vi "TwoCameraDisplayPanel.vi"() -> ()   [LabVIEW 2011]
uses:
  MvLVLib/MvCameraControl.lvlib
  MvLVLib/VIs/CreateGigEHandle.vi
  MvLVLib/VIs/CreateU3VHandle.vi
  <vilib>/picture/picture.llb/imagedata.ctl
panel:
  in  "image data 2":T1 caption="图像数据"
  in  "Rectangle 2":T2
  out "pFrameInfoEx out 2":T3
  in  "pConvertInfo In 2":T4
  out "nWidth 2":u32
  out "nHeight 2":u32
  out "PayloadSize 2":u32
  out "PixelFormat 2":u32
  out "handle out 2":u64
  in  "handle 2":u64
  out "Picture 2":picture
  in  "Device List 2":u16(ring)
  out "U3VDeviceArray":T5(array[cluster])
  out "GigEDeviceArray":T6(array[cluster])
  in  "pConvertInfo In":T4
  out "PixelFormat":u32
  out "handle out":u64
  in  "handle":u64
  in  "Rectangle":T2
  in  "image data":T1 caption="图像数据"
  out "Picture":picture
  out "PayloadSize":u32
  out "pFrameInfoEx out":T3
  out "nHeight":u32
  out "nWidth":u32
  out "Acquisision Flag":bool
  in  "Trigger Mode":bool
  in  "Continuous":bool
  out "打开标志":bool
  in  "stop":bool
  in  "Trigger Once":bool
  in  "Stop":bool
  in  "Start":bool
  in  "Open Device":bool
  in  "Close Device":bool
  in  "error in (no error) 2":errorcluster caption="错误输入（无错误）"
  in  "Refresh Devices":bool
  in  "Device List":u16(ring)
  # "Initialize"
  # "Acquisition"
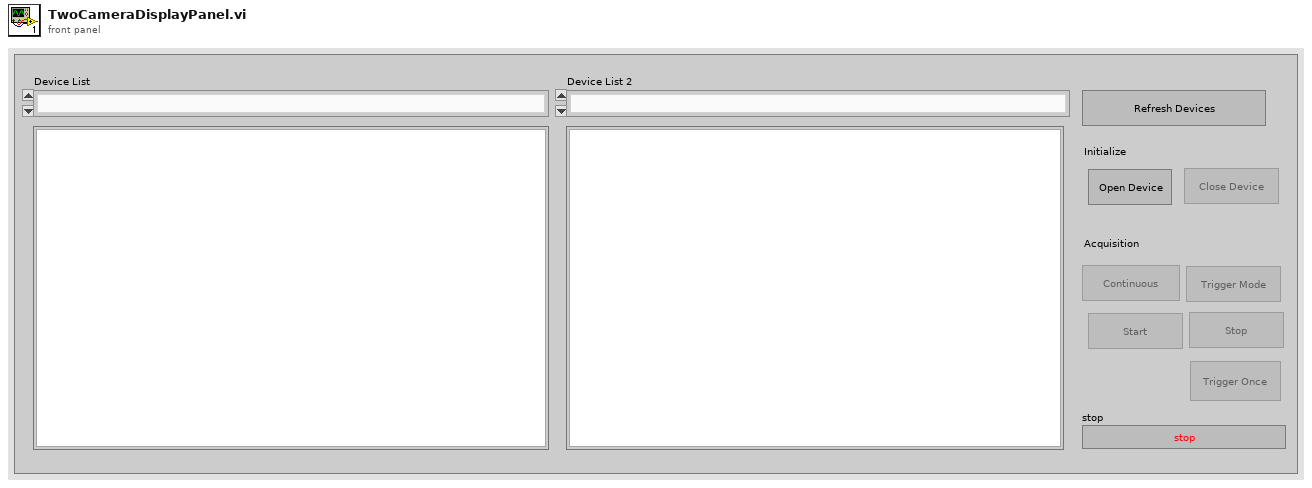
[diagram p1: front panel]
types:
  T1 = typedef "imagedata.ctl" = cluster{"image type":i32, "image depth":i32, "image":u8[], "mask":u8[], "colors":u32[], "Rectangle":cluster{"left":i16, "top":i16, "right":i16, "bottom":i16}}
  T2 = cluster{"left":i16, "top":i16, "right":i16, "bottom":i16}
  T3 = cluster{"nWidth":u16, "nHeight":u16, "enPixelType":i32, "nFrameNum":u32, "nDevTimeStampHigh":u32, "nDevTimeStampLow":u32, "nReserved0":u32, "nHostTimeStamp":i64, "nFrameLen":u32, "nSecondCount]":u32, "nCycleCount":u32, "nCycleOffset":u32, "fGain":u32, "fExposureTime":u32, "nAverageBrightness":u32, "nRed":u32, "nGreen":u32, "nBlue":u32, "nFrameCounter":u32, "nTriggerIndex":u32, "nInput":u32, "nOutput":u32, "nOffsetX":u32, "nOffsetY":u32, "nReserved[0]":u32, "nReserved[1]":u32, "nReserved[2]":u32, "nReserved[3]":u32, "nReserved[4]":u32, "nReserved[5]":u32, "nReserved[6]":u32, "nReserved[7]":u32, "nReserved[8]":u32, "nReserved[9]":u32, "nReserved[10]":u32, "nReserved[11]":u32, "nReserved[12]":u32, "nReserved[13]":u32, "nReserved[14] 10":u32, "nReserved[15] 11":u32, "nReserved[16] 12":u32, "nReserved[17] 13":u32, "nReserved[18] 14":u32, "nReserved[19] 15":u32, "nReserved[20] 16":u32, "nReserved[21] 17":u32, "nReserved[22] 18":u32, "nReserved[23] 19":u32, "nReserved[24] 20":u32, "nReserved[25] 21":u32, "nReserved[26] 22":u32, "nReserved[27] 23":u32, "nReserved[28] 24":u32, "nReserved[29] 25":u32, "nReserved[30] 26":u32, "nReserved[31] 27":u32, "nReserved[32] 28":u32, "nReserved[33] 29":u32, "nReserved[34] 30":u32, "nReserved[35] 31":u32, "nReserved[36] 32":u32, "nReserved[37] 33":u32, "nReserved[38] 34":u32, "nReserved[39] 35":u32, "nReserved[40] 36":u32}
  T4 = cluster{"nWidth":u16, "nHeight":u16, "enSrcPixelType":u32, "nSrcDataLen":u32, "enDstPixelType":u32, "nDstLen":u32, "nDstBufferSize":u32, "nRes0":u32, "nRes1":u32, "nRes2":u32, "nRes3":u32}
  T5 = cluster{"nMajorVer":u16, "nMinorVer":u16, "nMacAddrHigh":u32, "nMacAddrLow":u32, "nTLayerType":u32, "nReserved0":u32, "nReserved1":u32, "nReserved2":u32, "nReserved3":u32, "CrtlInEndPoint":u8, "CrtlOutEndPoint":u8, "StreamEndPoint":u8, "EventEndPoint":u8, "idVendor":u16, "idProduct":u16, "nDeviceNumber":u32, "chDeviceGUID":string, "chVendorName":string, "chModelName":string, "chFamilyName":string, "chDeviceVersion":string, "chManufacturerName":string, "chSerialNumber":string, "chUserDefinedName":string, "nbcdUSB":u32, "nDeviceAddress":u32, "nRes0":u32, "nRes1":u32, "nResAlign":u32}[]
  T6 = cluster{"nMajorVer":u16, "nMinorVer":u16, "nMacAddrHigh":u32, "nMacAddrLow":u32, "nTLayerType":u32, "nReserved0":u32, "nReserved1":u32, "nReserved2":u32, "nReserved3":u32, "nIpCfgOption":u32, "nIpCfgCurrent":u32, "nCurrentIp":u32, "nCurrentSubNetMask":u32, "nDefaultGateWay":u32, "chManualfacturerName":string, "chModelName":string, "chDeviceVersion":string, "chManufacturerSpecificInfo":string, "chSerialNumber":string, "chUserDefinedName":string, "nNetExport":u32, "nRes0":u32, "nRes1":u32, "nRes2":u32, "nRes3":u32}[]
  T7 = enum8{"Enabled", "Disabled", "Disabled and Grayed Out"}
  T8 = cluster{"nCurValue":u32, "nMax":u32, "nMin":u32, "nInc":u32, "nReserved[0]":u32, "nReserved[1]":u32, "nReserved[2]":u32, "nReserved[3]":u32}
  T9 = cluster{"nCurValue":u32, "nSupportedNum":u32, "nSupportValue[0]":u32, "nSupportValue[1]":u32, "nSupportValue[2]":u32, "nSupportValue[3]":u32, "nSupportValue[4]":u32, "nSupportValue[5]":u32, "nSupportValue[6]":u32, "nSupportValue[7]":u32, "nSupportValue[8]":u32, "nSupportValue[9]":u32, "nSupportValue[10]":u32, "nSupportValue[11]":u32, "nSupportValue[12]":u32, "nSupportValue[13]":u32, "nSupportValue[14]":u32, "nSupportValue[15]":u32, "nSupportValue[16]":u32, "nSupportValue[17]":u32, "nSupportValue[18]":u32, "nSupportValue[19]":u32, "nSupportValue[20]":u32, "nSupportValue[21]":u32, "nSupportValue[22]":u32, "nSupportValue[23]":u32, "nSupportValue[24]":u32, "nSupportValue[25]":u32, "nSupportValue[26]":u32, "nSupportValue[27]":u32, "nSupportValue[28]":u32, "nSupportValue[29]":u32, "nSupportValue[30]":u32, "nSupportValue[31]":u32, "nSupportValue[32]":u32, "nSupportValue[33]":u32, "nSupportValue[34]":u32, "nSupportValue[35]":u32, "nSupportValue[36]":u32, "nSupportValue[37]":u32, "nSupportValue[38]":u32, "nSupportValue[39]":u32, "nSupportValue[40]":u32, "nSupportValue[41]":u32, "nSupportValue[42]":u32, "nSupportValue[43]":u32, "nSupportValue[44]":u32, "nSupportValue[45]":u32, "nSupportValue[46]":u32, "nSupportValue[47]":u32, "nSupportValue[48]":u32, "nSupportValue[49]":u32, "nSupportValue[50]":u32, "nSupportValue[51]":u32, "nSupportValue[52]":u32, "nSupportValue[53]":u32, "nSupportValue[54]":u32, "nSupportValue[55]":u32, "nSupportValue[56]":u32, "nSupportValue[57]":u32, "nSupportValue[58]":u32, "nSupportValue[59]":u32, "nSupportValue[60]":u32, "nSupportValue[61]":u32, "nSupportValue[62]":u32, "nSupportValue[63]":u32, "nReserved[0]":u32, "nReserved[1]":u32, "nReserved[2]":u32, "nReserved[3]":u32}
  T10 = cluster{"nMajorVer":u16, "nMinorVer":u16, "nMacAddrHigh":u32, "nMacAddrLow":u32, "nTLayerType":u32, "nReserved0":u32, "nReserved1":u32, "nReserved2":u32, "nReserved3":u32, "CrtlInEndPoint":u8, "CrtlOutEndPoint":u8, "StreamEndPoint":u8, "EventEndPoint":u8, "idVendor":u16, "idProduct":u16, "nDeviceNumber":u32, "chDeviceGUID":string, "chVendorName":string, "chModelName":string, "chFamilyName":string, "chDeviceVersion":string, "chManufacturerName":string, "chSerialNumber":string, "chUserDefinedName":string, "nbcdUSB":u32, "nDeviceAddress":u32, "nRes0":u32, "nRes1":u32, "nResAlign":u32}
  T11 = cluster{"nMajorVer":u16, "nMinorVer":u16, "nMacAddrHigh":u32, "nMacAddrLow":u32, "nTLayerType":u32, "nReserved0":u32, "nReserved1":u32, "nReserved2":u32, "nReserved3":u32, "nIpCfgOption":u32, "nIpCfgCurrent":u32, "nCurrentIp":u32, "nCurrentSubNetMask":u32, "nDefaultGateWay":u32, "chManualfacturerName":string, "chModelName":string, "chDeviceVersion":string, "chManufacturerSpecificInfo":string, "chSerialNumber":string, "chUserDefinedName":string, "nNetExport":u32, "nRes0":u32, "nRes1":u32, "nRes2":u32, "nRes3":u32}
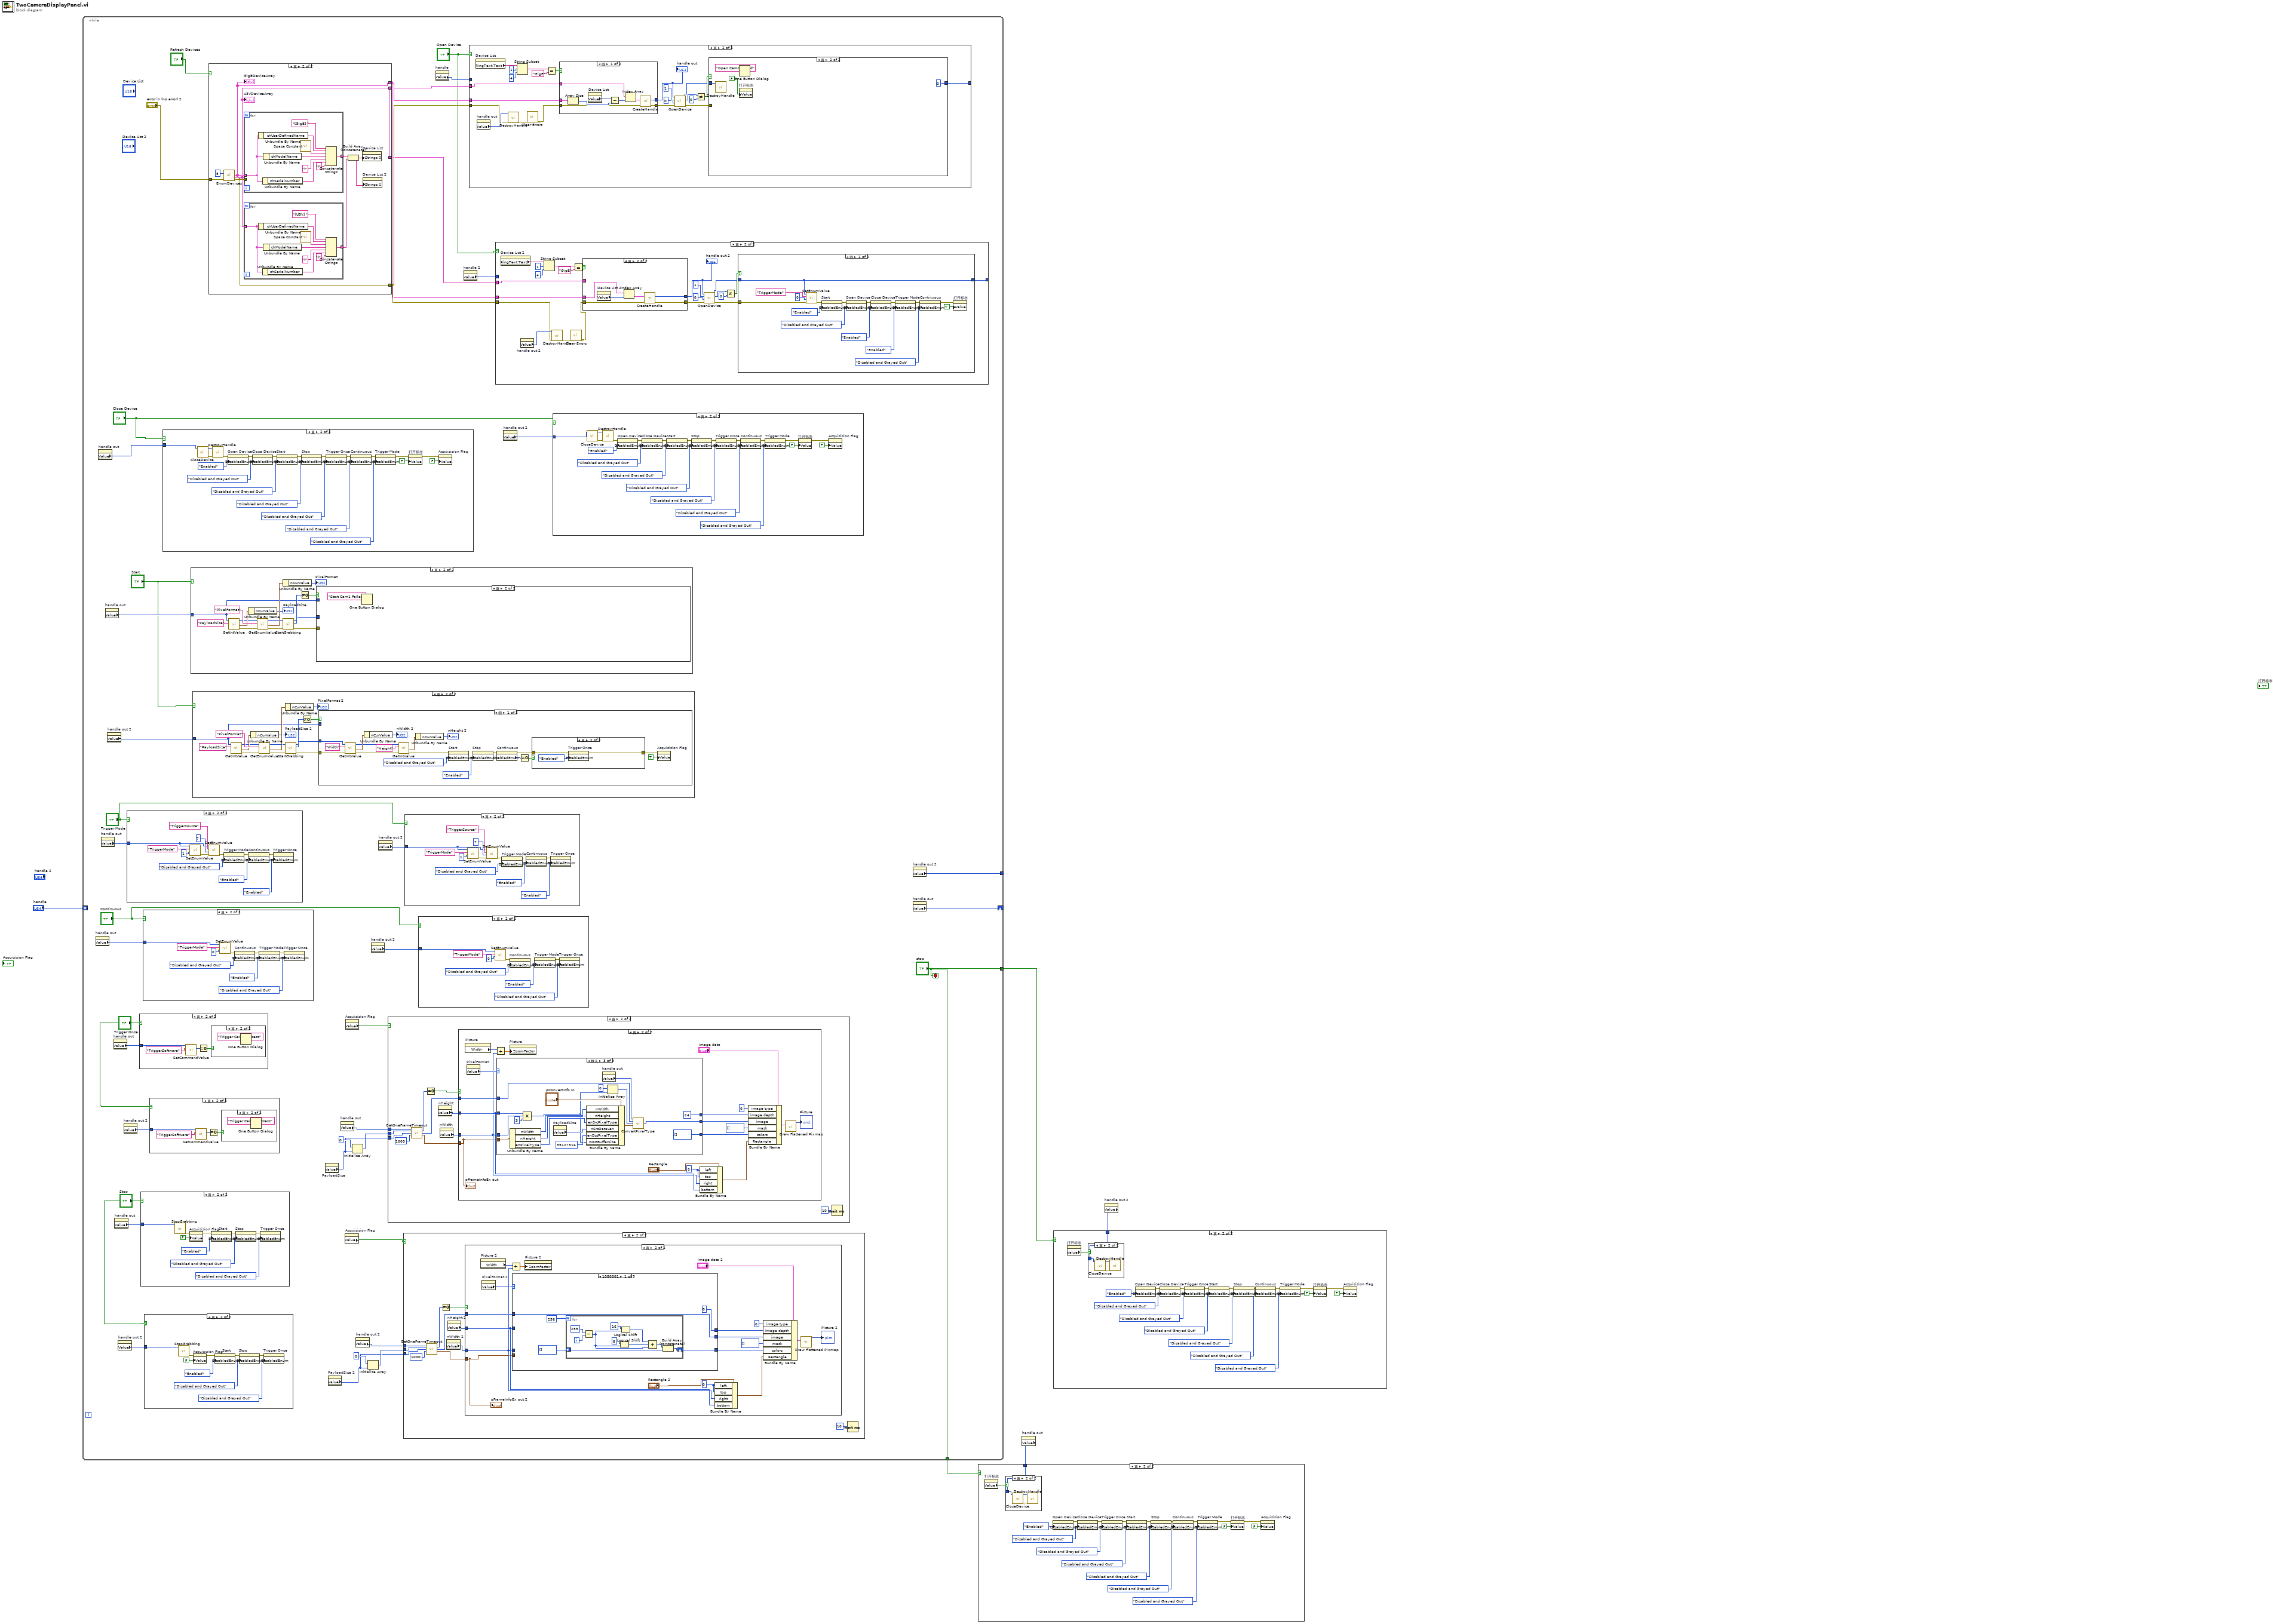
[diagram p0: block diagram]
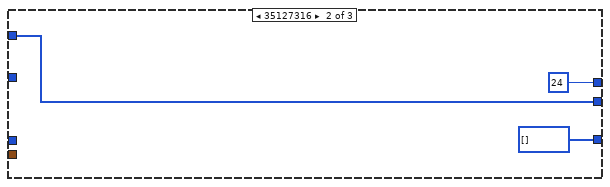
[diagram p8: hidden frame]
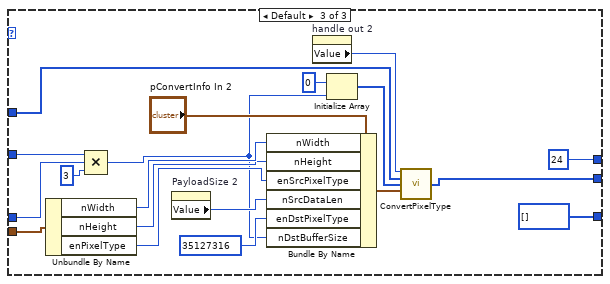
[diagram p9: hidden frame]
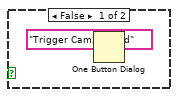
[diagram p11: hidden frame]
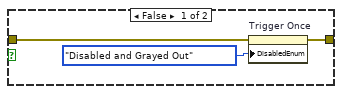
[diagram p16: hidden frame]
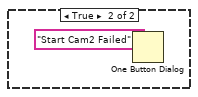
[diagram p17: hidden frame]
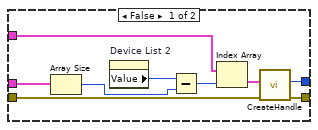
[diagram p20: hidden frame]
diagram:
  n1 = while {
    tunnel: ["stop"] -> w5
    shift-right: [w43] -> _
    shift-left: "handle" -> [_]
    tunnel: ["stop"] -> w1
    tunnel: [w9] -> _
    stop <- "stop" stop-if-true
    n2 = property on="handle out" class="DigNum (严格)"() -> ("Value"=w35:u64)  [unwired: 2 in, 2 out]
    n3 = property on="handle out" class="DigNum (严格)"() -> ("Value"=w41:u64)  [unwired: 2 in, 2 out]
    n4 = property on="handle out" class="DigNum (严格)"() -> ("Value"=w36:u64)  [unwired: 2 in, 2 out]
    n5 = property on="handle out" class="DigNum (严格)"() -> ("Value"=w37:u64)  [unwired: 2 in, 2 out]
    n6 = property on="handle out 2" class="DigNum (严格)"() -> ("Value"=w23:u64)  [unwired: 2 in, 2 out]
    n7 = property on="handle out" class="DigNum (严格)"() -> ("Value"=w40:u64)  [unwired: 2 in, 2 out]
    n8 = property on="handle out" class="DigNum (严格)"() -> ("Value"=w39:u64)  [unwired: 2 in, 2 out]
    n9 = property on="handle out 2" class="DigNum (严格)"() -> ("Value"=w17:u64)  [unwired: 2 in, 2 out]
    n10 = property on="handle out 2" class="DigNum (严格)"() -> ("Value"=w16:u64)  [unwired: 2 in, 2 out]
    n11 = case shown="真" "Trigger Mode" {
      tunnel: w36 -> [_ w350]
      frame False {
      }
      frame True {
        n12 = call "SetEnumValue.vi"("nValue"=u32 1, "strKey"="TriggerMode", "handle"=w350) -> ("error out"=w356:errorcluster)  [unwired: 6 in, 2 out]
        n13 = call "SetEnumValue.vi"("error in (no error)"=w356, "nValue"=u32 7, "strKey"="TriggerSource", "handle"=w350) -> ("error out"=w355:errorcluster)  [unwired: 5 in, 2 out]
        n14 = property on="Trigger Mode" class="Bool"(error in=w355, "DisabledEnum"=T7."Disabled and Grayed Out" ("禁用")) -> (error out=w354:errorcluster)  [unwired: 1 in, 1 out]
        n15 = property on="Continuous" class="Bool"(error in=w354, "DisabledEnum"=T7."Enabled" ("禁用")) -> (error out=w352:errorcluster)  [unwired: 1 in, 1 out]
        n16 = property on="Trigger Once" class="Bool"(error in=w352, "DisabledEnum"=T7."Enabled" ("禁用")) -> ()  [unwired: 1 in, 2 out]
      }
    }
    n17 = case shown="真" "Trigger Once" {
      tunnel: w40 -> [_ w365]
      frame False {
      }
      frame True {
        n18 = call "SetCommandValue.vi"("strValue"="TriggerSoftware", "handle"=w365) -> ("function return"=w363:i32)  [unwired: 7 in, 2 out]
        n19 = Equal To 0?(x=w363) -> (x = 0?=w362:bool)
        n20 = case shown="真" w362 {
          frame False {
            n21 = One Button Dialog(message="Trigger Cam1 Failed") -> ()  [unwired: 1 in, 1 out]
          }
          frame True {
            n22 = One Button Dialog(message="Trigger Can1 Success") -> ()  [unwired: 1 in, 1 out]
          }
        }
      }
    }
    n23 = case shown="真" "Stop" {
      tunnel: w39 -> [_ w340]
      frame False {
      }
      frame True {
        n24 = call "StopGrabbing.vi"("handle"=w340) -> ("error out"=w339:errorcluster)  [unwired: 8 in, 2 out]
        n25 = property on="Acquisision Flag" class="Bool (严格)"(error in=w339, "Value"=FALSE ("采集标志")) -> (error out=w334:errorcluster)  [unwired: 1 in, 1 out]
        n26 = property on="Start" class="Bool"(error in=w334, "DisabledEnum"=T7."Enabled" ("禁用")) -> (error out=w333:errorcluster)  [unwired: 1 in, 1 out]
        n27 = property on="Stop" class="Bool"(error in=w333, "DisabledEnum"=T7."Disabled and Grayed Out" ("禁用")) -> (error out=w332:errorcluster)  [unwired: 1 in, 1 out]
        n28 = property on="Trigger Once" class="Bool"(error in=w332, "DisabledEnum"=T7."Disabled and Grayed Out" ("禁用")) -> ()  [unwired: 1 in, 2 out]
      }
    }
    n29 = case shown="真" "Continuous" {
      tunnel: w35 -> [_ w341]
      frame False {
      }
      frame True {
        n30 = call "SetEnumValue.vi"("nValue"=u32 0, "strKey"="TriggerMode", "handle"=w341) -> ("error out"=w342:errorcluster)  [unwired: 6 in, 2 out]
        n31 = property on="Continuous" class="Bool"(error in=w342, "DisabledEnum"=T7."Disabled and Grayed Out" ("禁用")) -> (error out=w346:errorcluster)  [unwired: 1 in, 1 out]
        n32 = property on="Trigger Mode" class="Bool"(error in=w346, "DisabledEnum"=T7."Enabled" ("禁用")) -> (error out=w344:errorcluster)  [unwired: 1 in, 1 out]
        n33 = property on="Trigger Once" class="Bool"(error in=w344, "DisabledEnum"=T7."Disabled and Grayed Out" ("禁用")) -> ()  [unwired: 1 in, 2 out]
      }
    }
    n34 = case shown="真" "Stop" {
      tunnel: w17 -> [_ w126]
      frame False {
      }
      frame True {
        n35 = call "StopGrabbing.vi"("handle"=w126) -> ("error out"=w125:errorcluster)  [unwired: 8 in, 2 out]
        n36 = property on="Acquisision Flag" class="Bool (严格)"(error in=w125, "Value"=FALSE ("采集标志")) -> (error out=w120:errorcluster)  [unwired: 1 in, 1 out]
        n37 = property on="Start" class="Bool"(error in=w120, "DisabledEnum"=T7."Enabled" ("禁用")) -> (error out=w119:errorcluster)  [unwired: 1 in, 1 out]
        n38 = property on="Stop" class="Bool"(error in=w119, "DisabledEnum"=T7."Disabled and Grayed Out" ("禁用")) -> (error out=w118:errorcluster)  [unwired: 1 in, 1 out]
        n39 = property on="Trigger Once" class="Bool"(error in=w118, "DisabledEnum"=T7."Disabled and Grayed Out" ("禁用")) -> ()  [unwired: 1 in, 2 out]
      }
    }
    n40 = case shown="真" "Trigger Once" {
      tunnel: w16 -> [_ w115]
      frame False {
      }
      frame True {
        n41 = call "SetCommandValue.vi"("strValue"="TriggerSoftware", "handle"=w115) -> ("function return"=w113:i32)  [unwired: 7 in, 2 out]
        n42 = Equal To 0?(x=w113) -> (x = 0?=w112:bool)
        n43 = case shown="真" w112 {
          frame False {
            n44 = One Button Dialog(message="Trigger Cam2 Failed") -> ()  [unwired: 1 in, 1 out]
          }
          frame True {
            n45 = One Button Dialog(message="Trigger Cam2 Success") -> ()  [unwired: 1 in, 1 out]
          }
        }
      }
    }
    n46 = case shown="真" "Close Device" {
      tunnel: w41 -> [_ w411]
      frame False {
      }
      frame True {
        n47 = call "CloseDevice.vi"("handle"=w411) -> ("error out"=w413:errorcluster, "handle out"=w410:u64)  [unwired: 8 in, 1 out]
        n48 = call "DestroyHandle.vi"("error in (no error)"=w413, "handle"=w410) -> ("error out"=w412:errorcluster)  [unwired: 8 in, 1 out]
        n49 = property on="Open Device" class="Bool"(error in=w412, "DisabledEnum"=T7."Enabled" ("禁用")) -> (error out=w426:errorcluster)  [unwired: 1 in, 1 out]
        n50 = property on="Close Device" class="Bool"(error in=w426, "DisabledEnum"=T7."Disabled and Grayed Out" ("禁用")) -> (error out=w425:errorcluster)  [unwired: 1 in, 1 out]
        n51 = property on="Start" class="Bool"(error in=w425, "DisabledEnum"=T7."Disabled and Grayed Out" ("禁用")) -> (error out=w424:errorcluster)  [unwired: 1 in, 1 out]
        n52 = property on="Stop" class="Bool"(error in=w424, "DisabledEnum"=T7."Disabled and Grayed Out" ("禁用")) -> (error out=w423:errorcluster)  [unwired: 1 in, 1 out]
        n53 = property on="Trigger Once" class="Bool"(error in=w423, "DisabledEnum"=T7."Disabled and Grayed Out" ("禁用")) -> (error out=w420:errorcluster)  [unwired: 1 in, 1 out]
        n54 = property on="Continuous" class="Bool"(error in=w420, "DisabledEnum"=T7."Disabled and Grayed Out" ("禁用")) -> (error out=w418:errorcluster)  [unwired: 1 in, 1 out]
        n55 = property on="Trigger Mode" class="Bool"(error in=w418, "DisabledEnum"=T7."Disabled and Grayed Out" ("禁用")) -> (error out=w417:errorcluster)  [unwired: 1 in, 1 out]
        n56 = property on="打开标志" class="Bool (严格)"(error in=w417, "Value"=FALSE ("打开标志")) -> (error out=w415:errorcluster)  [unwired: 1 in, 1 out]
        n57 = property on="Acquisision Flag" class="Bool (严格)"(error in=w415, "Value"=FALSE ("采集标志")) -> ()  [unwired: 1 in, 2 out]
      }
    }
    n58 = case shown="真" "Start" {
      tunnel: w37 -> [_ w372]
      frame False {
      }
      frame True {
        n59 = call "GetIntValue.vi"("strKey"="PayloadSize", "handle"=w372) -> ("error out"=w378:errorcluster, "pIntValue out"=w374:T8, "handle out"=w370:u64)  [unwired: 6 in, 1 out]
        n60 = Unbundle By Name(w374) -> ("nCurValue"=→"PayloadSize":u32)
        n61 = call "GetEnumValue.vi"("error in (no error)"=w378, "strKey"="PixelFormat", "handle"=w370) -> ("error out"=w377:errorcluster, "pEnumValue out"=w379:T9, "handle out"=w369:u64)  [unwired: 5 in, 1 out]
        n62 = Unbundle By Name(w379) -> ("nCurValue"=→"PixelFormat":u32)
        n63 = call "StartGrabbing.vi"("error in (no error)"=w377, "handle"=w369) -> ("error out"=w376:errorcluster, "function return"=w382:i32, "handle out"=w368:u64)  [unwired: 7 in]
        n64 = Not Equal To 0?(x=w382) -> (x != 0?=w381:bool)
        n65 = case shown="真" w381 {
          tunnel: w372 -> [_ _]
          tunnel: w376 -> [w385 _]
          tunnel: w368 -> [w384 _]
          frame False {
            n66 = call "GetIntValue.vi"("error in (no error)"=w385, "strKey"="Width", "handle"=w384) -> ("error out"=w392:errorcluster, "pIntValue out"=w386:T8, "handle out"=w383:u64)  [unwired: 5 in, 1 out]
            n67 = Unbundle By Name(w386) -> ("nCurValue"=→"nWidth":u32)
            n68 = call "GetIntValue.vi"("error in (no error)"=w392, "strKey"="Height", "handle"=w383) -> ("error out"=w391:errorcluster, "pIntValue out"=w389:T8)  [unwired: 5 in, 2 out]
            n69 = Unbundle By Name(w389) -> ("nCurValue"=→"nHeight":u32)
            n70 = property on="Start" class="Bool"(error in=w391, "DisabledEnum"=T7."Disabled and Grayed Out" ("禁用")) -> (error out=w401:errorcluster)  [unwired: 1 in, 1 out]
            n71 = property on="Stop" class="Bool"(error in=w401, "DisabledEnum"=T7."Enabled" ("禁用")) -> (error out=w387:errorcluster)  [unwired: 1 in, 1 out]
            n72 = property on="Continuous" class="Bool"(error in=w387) -> (error out=w397:errorcluster, "DisabledEnum"=w398:T7)  [unwired: 1 in, 1 out]
            n73 = Equal To 0?(x=w398) -> (x = 0?=w399:bool)
            n74 = case shown="真" w399 {
              tunnel: w397 -> [w404 w407]
              tunnel: [w403 w406] -> w396
              frame False {
                n75 = property on="Trigger Once" class="Bool"(error in=w404, "DisabledEnum"=T7."Disabled and Grayed Out" ("禁用")) -> (error out=w403:errorcluster)  [unwired: 1 in, 1 out]
              }
              frame True {
                n76 = property on="Trigger Once" class="Bool"(error in=w407, "DisabledEnum"=T7."Enabled" ("禁用")) -> (error out=w406:errorcluster)  [unwired: 1 in, 1 out]
              }
            }
            n77 = property on="Acquisision Flag" class="Bool (严格)"(error in=w396, "Value"=TRUE ("采集标志")) -> ()  [unwired: 1 in, 2 out]
          }
          frame True {
            n78 = One Button Dialog(message="Start Cam1 Failed") -> ()  [unwired: 1 in, 1 out]
          }
        }
      }
    }
    n79 = case shown="真" "Start" {
      tunnel: w23 -> [_ w150]
      frame False {
      }
      frame True {
        n80 = call "GetIntValue.vi"("strKey"="PayloadSize", "handle"=w150) -> ("error out"=w156:errorcluster, "pIntValue out"=w152:T8, "handle out"=w148:u64)  [unwired: 6 in, 1 out]
        n81 = Unbundle By Name(w152) -> ("nCurValue"=→"PayloadSize 2":u32)
        n82 = call "GetEnumValue.vi"("error in (no error)"=w156, "strKey"="PixelFormat", "handle"=w148) -> ("error out"=w155:errorcluster, "pEnumValue out"=w157:T9, "handle out"=w147:u64)  [unwired: 5 in, 1 out]
        n83 = Unbundle By Name(w157) -> ("nCurValue"=→"PixelFormat 2":u32)
        n84 = call "StartGrabbing.vi"("error in (no error)"=w155, "handle"=w147) -> ("error out"=w154:errorcluster, "function return"=w160:i32, "handle out"=w146:u64)  [unwired: 7 in]
        n85 = Not Equal To 0?(x=w160) -> (x != 0?=w159:bool)
        n86 = case shown="假" w159 {
          tunnel: w150 -> [_ _]
          tunnel: w154 -> [w165 _]
          tunnel: w146 -> [w164 _]
          frame False {
            n87 = call "GetIntValue.vi"("error in (no error)"=w165, "strKey"="Width", "handle"=w164) -> ("error out"=w171:errorcluster, "pIntValue out"=w166:T8, "handle out"=w163:u64)  [unwired: 5 in, 1 out]
            n88 = Unbundle By Name(w166) -> ("nCurValue"=→"nWidth 2":u32)
            n89 = call "GetIntValue.vi"("error in (no error)"=w171, "strKey"="Height", "handle"=w163) -> ("error out"=w162:errorcluster, "pIntValue out"=w169:T8)  [unwired: 5 in, 2 out]
            n90 = Unbundle By Name(w169) -> ("nCurValue"=→"nHeight 2":u32)
            n91 = property on="Start" class="Bool"(error in=w162, "DisabledEnum"=T7."Disabled and Grayed Out" ("禁用")) -> ()  [unwired: 1 in, 2 out]
            n92 = property on="Stop" class="Bool"("DisabledEnum"=T7."Enabled" ("禁用")) -> (error out=w167:errorcluster)  [unwired: 2 in, 1 out]
            n93 = property on="Continuous" class="Bool"(error in=w167) -> (error out=w176:errorcluster, "DisabledEnum"=w177:T7)  [unwired: 1 in, 1 out]
            n94 = Equal To 0?(x=w177) -> (x = 0?=w178:bool)
            n95 = case shown="真" w178 {
              tunnel: w176 -> [w181 w184]
              tunnel: [w180 w183] -> w175
              frame False {
                n96 = property on="Trigger Once" class="Bool"(error in=w181, "DisabledEnum"=T7."Disabled and Grayed Out" ("禁用")) -> (error out=w180:errorcluster)  [unwired: 1 in, 1 out]
              }
              frame True {
                n97 = property on="Trigger Once" class="Bool"(error in=w184, "DisabledEnum"=T7."Enabled" ("禁用")) -> (error out=w183:errorcluster)  [unwired: 1 in, 1 out]
              }
            }
            n98 = property on="Acquisision Flag" class="Bool (严格)"(error in=w175, "Value"=TRUE ("采集标志")) -> ()  [unwired: 1 in, 2 out]
          }
          frame True {
            n99 = One Button Dialog(message="Start Cam2 Failed") -> ()  [unwired: 1 in, 1 out]
          }
        }
      }
    }
    n100 = case shown="真" "Refresh Devices" {
      tunnel: [w491 w498] -> w30
      tunnel: "error in (no error) 2" -> [w491 w497]
      tunnel: [w489 w492] -> w31
      tunnel: [w490 w494] -> w29
      tunnel: [w489 w492] -> w28
      frame False {
        n101 = property on="U3VDeviceArray" class="Arr (严格)"() -> ("Value"=w489:T5)  [unwired: 2 in, 2 out]
        n102 = property on="GigEDeviceArray" class="Arr (严格)"() -> ("Value"=w490:T6)  [unwired: 2 in, 2 out]
      }
      frame True {
        n103 = call "EnumDevices.vi"("nLayerType"=u32 5, "error in (no error)"=w497) -> ("GigEDeviceArray"=w494:T6, "U3VDeviceArray"=w492:T5, "error out"=w498:errorcluster)  [unwired: 9 in, 2 out]
        "GigEDeviceArray" <- w494
        "U3VDeviceArray" <- w492
        n104 = for {
          tunnel: w498 -> [_]
          tunnel: w494 -> [w511] mode=indexing
          tunnel: [w510] -> w496 mode=indexing
          n105 = Unbundle By Name(w511) -> ("chUserDefinedName"=w514:string)
          n106 = Unbundle By Name(w511) -> ("chSerialNumber"=w512:string)
          n107 = Unbundle By Name(w511) -> ("chModelName"=w513:string)
          n108 = call <vilib>:"Space Constant.vi"() -> ("String"=w517:string)
          n109 = Concatenate Strings("[GigE] " ("字符串"), w514, w517, w513, "(" ("字符串"), w512, ")" ("字符串")) -> (w510:string)
        }
        n110 = for {
          tunnel: w492 -> [w504] mode=indexing
          tunnel: [w501] -> w495 mode=indexing
          n111 = Unbundle By Name(w504) -> ("chUserDefinedName"=w508:string)
          n112 = Unbundle By Name(w504) -> ("chSerialNumber"=w503:string)
          n113 = Unbundle By Name(w504) -> ("chModelName"=w506:string)
          n114 = call <vilib>:"Space Constant.vi"() -> ("String"=w507:string)
          n115 = Concatenate Strings("[U3V] " ("字符串"), w508, w507, w506, "(" ("字符串"), w503, ")" ("字符串")) -> (w501:string)
        }
        n116 = Build Array (concatenate)(w496, w495) -> (w493:string[])
        n117 = property on="Device List" class="Ring (严格)"("Strings []"=w493) -> ()  [unwired: 2 in, 2 out]
        n118 = property on="Device List 2" class="Ring (严格)"("Strings []"=w493) -> ()  [unwired: 2 in, 2 out]
      }
    }
    n119 = property on="PayloadSize" class="DigNum (严格)"() -> ("Value"=w32:u32)  [unwired: 2 in, 2 out]
    n120 = property on="PayloadSize 2" class="DigNum (严格)"() -> ("Value"=w11:u32)  [unwired: 2 in, 2 out]
    n121 = property on="handle out" class="DigNum (严格)"() -> ("Value"=w38:u64)  [unwired: 2 in, 2 out]
    n122 = property on="Acquisision Flag" class="Bool (严格)"() -> ("Value"=w7:bool)  [unwired: 2 in, 2 out]
    n123 = property on="Acquisision Flag" class="Bool (严格)"() -> ("Value"=w8:bool)  [unwired: 2 in, 2 out]
    n124 = Initialize Array(u8 0 ("元素"), w32) -> (w33:u8[])
    n125 = property on="handle out 2" class="DigNum (严格)"() -> ("Value"=w14:u64)  [unwired: 2 in, 2 out]
    n126 = Initialize Array(u8 0 ("元素"), w11) -> (w12:u8[])
    n127 = property on="handle out 2" class="DigNum (严格)"() -> ("Value"=w19:u64)  [unwired: 2 in, 2 out]
    n128 = property on="handle out 2" class="DigNum (严格)"() -> ("Value"=w21:u64)  [unwired: 2 in, 2 out]
    n129 = case shown="真" w8 {
      tunnel: w38 -> [_ w271]
      tunnel: w33 -> [_ w270]
      tunnel: w32 -> [_ w269]
      frame False {
      }
      frame True {
        n130 = call "GetOneFrameTimeout.vi"("handle"=w271, "pData"=w270, "nDataSize"=w269, "nMsec"=1000) -> ("function return"=w268:i32, "pData Out"=w267:u8[], "pFrameInfoEx out"=w266:T3)  [unwired: 7 in, 2 out]
        n131 = Equal To 0?(x=w268) -> (x = 0?=w275:bool)
        n132 = property on="nHeight" class="DigNum (严格)"() -> ("Value"=w273:u32)  [unwired: 2 in, 2 out]
        n133 = property on="nWidth" class="DigNum (严格)"() -> ("Value"=w274:u32)  [unwired: 2 in, 2 out]
        n134 = case shown="真" w275 {
          tunnel: w267 -> [_ w284]
          tunnel: w274 -> [_ w282]
          tunnel: w273 -> [_ w283]
          tunnel: w266 -> [_ w278]
          frame False {
          }
          frame True {
            w291 = i16 0 ("left")
            n135 = property on="Picture" class="Pict"() -> ("Width"=w286:u32)  [unwired: 2 in, 2 out]
            n136 = property on="PixelFormat" class="DigNum (严格)"() -> ("Value"=w279:u32)  [unwired: 2 in, 2 out]
            n137 = Divide(x=w286, y=w282) -> (x/y=w285:dbl)
            n138 = case shown="默认" w279 {
              tunnel: w284 -> [w297 w312 w328]
              tunnel: w283 -> [_ _ w325]
              tunnel: w282 -> [_ _ w324]
              tunnel: [w297 w312 w313] -> w281
              tunnel: [8 24 24] -> w277
              tunnel: [w295 i32[] [] i32[] []] -> w280
              tunnel: w278 -> [_ _ w314]
              frame 17301505 {
                n139 = for {
                  N: 256 -> [_]
                  shift-right: [w304] -> w295
                  shift-left: i32[] [] ("数组") -> [w303]
                  i -> [w300]
                  n140 = Subtract(x=255, y=w300) -> (x-y=w301:i32)
                  n141 = Logical Shift(y=i16 8, x=w301) -> (x << y=w306:i32)
                  n142 = Logical Shift(y=16 ("x"), x=w301) -> (x << y=w307:i32)
                  n143 = Compound Arithmetic op=ADD(w307, w306, w301) -> (w305:i32)
                  n144 = Build Array (concatenate)(w305, w303) -> (w304:i32[])
                }
              }
              frame 35127316 {
              }
              frame Default {
                n145 = Unbundle By Name(w314) -> ("nWidth"=w323:u16, "nHeight"=w322:u16, "enPixelType"=w321:i32)
                n146 = Compound Arithmetic op=MULTIPLY(w325, w324, u32 3 ("值")) -> (w318:u32)
                n147 = property on="PayloadSize" class="DigNum (严格)"() -> ("Value"=w320:u32)  [unwired: 2 in, 2 out]
                n148 = Bundle By Name(cluster="pConvertInfo In", "nWidth"=w323, "nHeight"=w322, "enSrcPixelType"=w321, "nSrcDataLen"=w320, "enDstPixelType"=u32 35127316, "nDstBufferSize"=w318) -> (w317:T4)
                n149 = property on="handle out" class="DigNum (严格)"() -> ("Value"=w329:u64)  [unwired: 2 in, 2 out]
                n150 = Initialize Array(u8 0 ("元素"), w318) -> (w327:u8[])
                n151 = call "ConvertPixelType.vi"("handle"=w329, "pSrcData"=w328, "pDstBuf In"=w327, "pConvertInfo In"=w317) -> ("pDstBuf Out"=w313:u8[])  [unwired: 7 in, 4 out]
              }
            }
            n152 = property on="Picture" class="Pict"("ZoomFactor"=w285) -> ()  [unwired: 2 in, 2 out]
            n153 = Bundle By Name(cluster="Rectangle", "left"=w291, "top"=w291, "right"=w282, "bottom"=w283) -> (w288:T2)
            n154 = Bundle By Name(cluster="image data", "image type"=0, "image depth"=w277, "image"=w281, "mask"=u8[] [], "colors"=w280, "Rectangle"=w288) -> (w287:T1)
            n155 = call <vilib>:"Draw Flattened Pixmap.vi"("image data"=w287) -> ("new picture"=→"Picture":picture)  [unwired: 8 in]
            "pFrameInfoEx out" <- w278
          }
        }
        n156 = Wait (ms)(milliseconds to wait=u32 10 ("等待时间（毫秒）")) -> ()  [unwired: 1 out]
      }
    }
    n157 = case shown="真" w7 {
      tunnel: w14 -> [_ w51]
      tunnel: w12 -> [_ w50]
      tunnel: w11 -> [_ w49]
      frame False {
      }
      frame True {
        n158 = call "GetOneFrameTimeout.vi"("handle"=w51, "pData"=w50, "nDataSize"=w49, "nMsec"=1000) -> ("function return"=w48:i32, "pData Out"=w47:u8[], "pFrameInfoEx out"=w46:T3)  [unwired: 7 in, 2 out]
        n159 = Equal To 0?(x=w48) -> (x = 0?=w55:bool)
        n160 = property on="nWidth 2" class="DigNum (严格)"() -> ("Value"=w54:u32)  [unwired: 2 in, 2 out]
        n161 = property on="nHeight 2" class="DigNum (严格)"() -> ("Value"=w53:u32)  [unwired: 2 in, 2 out]
        n162 = case shown="真" w55 {
          tunnel: w47 -> [_ w67]
          tunnel: w54 -> [_ w65]
          tunnel: w53 -> [_ w66]
          tunnel: w46 -> [_ w60]
          frame False {
          }
          frame True {
            w74 = i16 0 ("left")
            n163 = property on="Picture 2" class="Pict"() -> ("Width"=w69:u32)  [unwired: 2 in, 2 out]
            n164 = property on="PixelFormat 2" class="DigNum (严格)"() -> ("Value"=w62:u32)  [unwired: 2 in, 2 out]
            n165 = Divide(x=w69, y=w65) -> (x/y=w68:dbl)
            n166 = case shown="1080001" w62 {
              tunnel: w67 -> [w77 w92 w108]
              tunnel: w66 -> [_ _ w105]
              tunnel: w65 -> [_ _ w104]
              tunnel: [w77 w92 w93] -> w64
              tunnel: [8 24 24] -> w57
              tunnel: [w75 i32[] [] i32[] []] -> w63
              tunnel: w60 -> [_ _ w94]
              frame 17301505 {
                n167 = for {
                  N: 256 -> [_]
                  shift-right: [w84] -> w75
                  shift-left: i32[] [] ("数组") -> [w83]
                  i -> [w80]
                  n168 = Subtract(x=255, y=w80) -> (x-y=w81:i32)
                  n169 = Logical Shift(y=i16 8, x=w81) -> (x << y=w86:i32)
                  n170 = Logical Shift(y=16 ("x"), x=w81) -> (x << y=w87:i32)
                  n171 = Compound Arithmetic op=ADD(w87, w86, w81) -> (w85:i32)
                  n172 = Build Array (concatenate)(w85, w83) -> (w84:i32[])
                }
              }
              frame 35127316 {
              }
              frame Default {
                n173 = Unbundle By Name(w94) -> ("nWidth"=w103:u16, "nHeight"=w102:u16, "enPixelType"=w101:i32)
                n174 = Compound Arithmetic op=MULTIPLY(w105, w104, u32 3 ("值")) -> (w98:u32)
                n175 = property on="PayloadSize 2" class="DigNum (严格)"() -> ("Value"=w100:u32)  [unwired: 2 in, 2 out]
                n176 = Bundle By Name(cluster="pConvertInfo In 2", "nWidth"=w103, "nHeight"=w102, "enSrcPixelType"=w101, "nSrcDataLen"=w100, "enDstPixelType"=u32 35127316, "nDstBufferSize"=w98) -> (w97:T4)
                n177 = property on="handle out 2" class="DigNum (严格)"() -> ("Value"=w109:u64)  [unwired: 2 in, 2 out]
                n178 = Initialize Array(u8 0 ("元素"), w98) -> (w107:u8[])
                n179 = call "ConvertPixelType.vi"("handle"=w109, "pSrcData"=w108, "pDstBuf In"=w107, "pConvertInfo In"=w97) -> ("pDstBuf Out"=w93:u8[])  [unwired: 7 in, 4 out]
              }
            }
            n180 = property on="Picture 2" class="Pict"("ZoomFactor"=w68) -> ()  [unwired: 2 in, 2 out]
            n181 = Bundle By Name(cluster="Rectangle 2", "left"=w74, "top"=w74, "right"=w65, "bottom"=w66) -> (w71:T2)
            n182 = Bundle By Name(cluster="image data 2", "image type"=0, "image depth"=w57, "image"=w64, "mask"=u8[] [], "colors"=w63, "Rectangle"=w71) -> (w70:T1)
            n183 = call <vilib>:"Draw Flattened Pixmap.vi"("image data"=w70) -> ("new picture"=→"Picture 2":picture)  [unwired: 8 in]
            "pFrameInfoEx out 2" <- w60
          }
        }
        n184 = Wait (ms)(milliseconds to wait=u32 10 ("等待时间（毫秒）")) -> ()  [unwired: 1 out]
      }
    }
    n185 = case shown="真" "Trigger Mode" {
      tunnel: w21 -> [_ w137]
      frame False {
      }
      frame True {
        n186 = call "SetEnumValue.vi"("nValue"=u32 1, "strKey"="TriggerMode", "handle"=w137) -> ("error out"=w141:errorcluster)  [unwired: 6 in, 2 out]
        n187 = call "SetEnumValue.vi"("error in (no error)"=w141, "nValue"=u32 7, "strKey"="TriggerSource", "handle"=w137) -> ("error out"=w136:errorcluster)  [unwired: 5 in, 2 out]
        n188 = property on="Trigger Mode" class="Bool"(error in=w136, "DisabledEnum"=T7."Disabled and Grayed Out" ("禁用")) -> ()  [unwired: 1 in, 2 out]
        n189 = property on="Continuous" class="Bool"("DisabledEnum"=T7."Enabled" ("禁用")) -> (error out=w139:errorcluster)  [unwired: 2 in, 1 out]
        n190 = property on="Trigger Once" class="Bool"(error in=w139, "DisabledEnum"=T7."Enabled" ("禁用")) -> ()  [unwired: 1 in, 2 out]
      }
    }
    n191 = case shown="真" "Continuous" {
      tunnel: w19 -> [_ w129]
      frame False {
      }
      frame True {
        n192 = call "SetEnumValue.vi"("nValue"=u32 0, "strKey"="TriggerMode", "handle"=w129) -> ("error out"=w128:errorcluster)  [unwired: 6 in, 2 out]
        n193 = property on="Continuous" class="Bool"(error in=w128, "DisabledEnum"=T7."Disabled and Grayed Out" ("禁用")) -> ()  [unwired: 1 in, 2 out]
        n194 = property on="Trigger Mode" class="Bool"("DisabledEnum"=T7."Enabled" ("禁用")) -> (error out=w131:errorcluster)  [unwired: 2 in, 1 out]
        n195 = property on="Trigger Once" class="Bool"(error in=w131, "DisabledEnum"=T7."Disabled and Grayed Out" ("禁用")) -> ()  [unwired: 1 in, 2 out]
      }
    }
    n196 = property on="handle" class="DigNum (严格)"() -> ("Value"=w42:u64)  [unwired: 2 in, 2 out]
    n197 = property on="handle 2" class="DigNum (严格)"() -> ("Value"=w27:u64)  [unwired: 2 in, 2 out]
    n198 = case shown="真" "Open Device" {
      tunnel: [w431 w446] -> _
      tunnel: w42 -> [w431 _]
      tunnel: w30 -> [_ w433]
      tunnel: w31 -> [_ w437]
      tunnel: w29 -> [_ w436]
      frame False {
      }
      frame True {
        n199 = property on="Device List" class="Ring (严格)"() -> ("RingText.Text"=w445:string)  [unwired: 2 in, 2 out]
        n200 = property on="handle out" class="DigNum (严格)"() -> ("Value"=w435:u64)  [unwired: 2 in, 2 out]
        n201 = call "DestroyHandle.vi"("error in (no error)"=w433, "handle"=w435) -> ("error out"=w434:errorcluster)  [unwired: 8 in, 1 out]
        n202 = String Subset(string=w445, offset (0)=1 ("偏移量(0)"), length (rest)=4 ("长度（剩余）")) -> (substring=w442:string)
        n203 = call <vilib>:"Clear Errors.vi"("error in (no error)"=w434) -> ("error out"=w432:errorcluster)  [unwired: 5 in, 1 out]
        n204 = Equal?(x=w442, y="GigE") -> (x = y?=w441:bool)
        n205 = case shown="假" w441 {
          tunnel: [w456 w465] -> w451
          tunnel: [w455 w464] -> w447
          tunnel: w436 -> [w460 w467]
          tunnel: w432 -> [w457 w466]
          tunnel: w437 -> [w462 _]
          frame False {
            n206 = Array Size(array=w460) -> (size(s)=w459:i32)
            n207 = property on="Device List" class="Ring (严格)"() -> ("Value"=w461:u16)  [unwired: 2 in, 2 out]
            n208 = Subtract(x=w461, y=w459) -> (x-y=w458:i32)
            n209 = Index Array(array=w462, index=w458) -> (element=w454:T10)
            n210 = call-poly "CreateHandle.vi"("error in (no error)"=w457, "U3VDevice"=w454) -> ("error out"=w456:errorcluster, "handle"=w455:u64)  [unwired: 6 in, 1 out]
          }
          frame True {
            n211 = property on="Device List" class="Ring (严格)"() -> ("Value"=w468:u16)  [unwired: 2 in, 2 out]
            n212 = Index Array(array=w467, index=w468) -> (element=w463:T11)
            n213 = call-poly "CreateHandle.vi"("error in (no error)"=w466, "GigEDevice"=w463) -> ("error out"=w465:errorcluster, "handle"=w464:u64)  [unwired: 6 in, 1 out]
          }
        }
        "handle out" <- w447
        n214 = call "OpenDevice.vi"("error in (no error)"=w451, "nSwitchoverKey"=u16 0, "nAccessMode"=u32 1, "handle"=w447) -> ("error out"=w448:errorcluster, "return"=w439:i32, "handle out"=w438:u64)  [unwired: 5 in]
        n215 = Not Equal?(x=w439, y=0) -> (x != y?=w452:bool)
        n216 = case shown="真" w452 {
          tunnel: w438 -> [w469 w486]
          tunnel: w448 -> [w470 _]
          tunnel: [w469 u64 0 ("handle")] -> w446
          frame False {
            n217 = call "SetEnumValue.vi"("error in (no error)"=w470, "nValue"=u32 0, "strKey"="TriggerMode", "handle"=w469) -> ("error out"=w481:errorcluster)  [unwired: 5 in, 2 out]
            n218 = property on="Start" class="Bool"(error in=w481, "DisabledEnum"=T7."Enabled" ("禁用")) -> (error out=w479:errorcluster)  [unwired: 1 in, 1 out]
            n219 = property on="Open Device" class="Bool"(error in=w479, "DisabledEnum"=T7."Disabled and Grayed Out" ("禁用")) -> (error out=w478:errorcluster)  [unwired: 1 in, 1 out]
            n220 = property on="Close Device" class="Bool"(error in=w478, "DisabledEnum"=T7."Enabled" ("禁用")) -> (error out=w475:errorcluster)  [unwired: 1 in, 1 out]
            n221 = property on="Trigger Mode" class="Bool"(error in=w475, "DisabledEnum"=T7."Enabled" ("禁用")) -> (error out=w473:errorcluster)  [unwired: 1 in, 1 out]
            n222 = property on="Continuous" class="Bool"(error in=w473, "DisabledEnum"=T7."Disabled and Grayed Out" ("禁用")) -> (error out=w471:errorcluster)  [unwired: 1 in, 1 out]
            n223 = property on="打开标志" class="Bool (严格)"(error in=w471, "Value"=TRUE ("布尔")) -> ()  [unwired: 1 in, 2 out]
          }
          frame True {
            n224 = call "DestroyHandle.vi"("handle"=w486) -> ()  [unwired: 9 in, 2 out]
            n225 = One Button Dialog(message="Open Cam1 Failed") -> ()  [unwired: 1 in, 1 out]
            n226 = property on="打开标志" class="Bool (严格)"("Value"=FALSE) -> ()  [unwired: 2 in, 2 out]
          }
        }
      }
    }
    n227 = case shown="真" "Open Device" {
      tunnel: [w208 w224] -> _
      tunnel: w27 -> [w208 _]
      tunnel: w30 -> [_ w210]
      tunnel: w28 -> [_ w216]
      tunnel: w29 -> [_ w215]
      frame False {
      }
      frame True {
        n228 = property on="Device List 2" class="Ring (严格)"() -> ("RingText.Text"=w214:string)  [unwired: 2 in, 2 out]
        n229 = property on="handle out 2" class="DigNum (严格)"() -> ("Value"=w211:u64)  [unwired: 2 in, 2 out]
        n230 = String Subset(string=w214, offset (0)=1 ("偏移量(0)"), length (rest)=4 ("长度（剩余）")) -> (substring=w221:string)
        n231 = call "DestroyHandle.vi"("error in (no error)"=w210, "handle"=w211) -> ("error out"=w212:errorcluster)  [unwired: 8 in, 1 out]
        n232 = call <vilib>:"Clear Errors.vi"("error in (no error)"=w212) -> ("error out"=w209:errorcluster)  [unwired: 5 in, 1 out]
        n233 = Equal?(x=w221, y="GigE") -> (x = y?=w220:bool)
        n234 = case shown="真" w220 {
          tunnel: [w233 w243] -> w228
          tunnel: [w232 w242] -> w213
          tunnel: w215 -> [w237 w245]
          tunnel: w209 -> [w234 w244]
          tunnel: w216 -> [w239 _]
          frame False {
            n235 = Array Size(array=w237) -> (size(s)=w236:i32)
            n236 = property on="Device List 2" class="Ring (严格)"() -> ("Value"=w238:u16)  [unwired: 2 in, 2 out]
            n237 = Subtract(x=w238, y=w236) -> (x-y=w235:i32)
            n238 = Index Array(array=w239, index=w235) -> (element=w231:T10)
            n239 = call-poly "CreateHandle.vi"("error in (no error)"=w234, "U3VDevice"=w231) -> ("error out"=w233:errorcluster, "handle"=w232:u64)  [unwired: 6 in, 1 out]
          }
          frame True {
            n240 = property on="Device List 2" class="Ring (严格)"() -> ("Value"=w240:u16)  [unwired: 2 in, 2 out]
            n241 = Index Array(array=w245, index=w240) -> (element=w241:T11)
            n242 = call-poly "CreateHandle.vi"("error in (no error)"=w244, "GigEDevice"=w241) -> ("error out"=w243:errorcluster, "handle"=w242:u64)  [unwired: 6 in, 1 out]
          }
        }
        "handle out 2" <- w213
        n243 = call "OpenDevice.vi"("error in (no error)"=w228, "nSwitchoverKey"=u16 0, "nAccessMode"=u32 1, "handle"=w213) -> ("error out"=w225:errorcluster, "return"=w218:i32, "handle out"=w217:u64)  [unwired: 5 in]
        n244 = Not Equal?(x=w218, y=0) -> (x != y?=w229:bool)
        n245 = case shown="假" w229 {
          tunnel: w217 -> [w246 w263]
          tunnel: w225 -> [w247 _]
          tunnel: [w246 u64 0 ("handle")] -> w224
          frame False {
            n246 = call "SetEnumValue.vi"("error in (no error)"=w247, "nValue"=u32 0, "strKey"="TriggerMode", "handle"=w246) -> ("error out"=w258:errorcluster)  [unwired: 5 in, 2 out]
            n247 = property on="Start" class="Bool"(error in=w258, "DisabledEnum"=T7."Enabled" ("禁用")) -> (error out=w256:errorcluster)  [unwired: 1 in, 1 out]
            n248 = property on="Open Device" class="Bool"(error in=w256, "DisabledEnum"=T7."Disabled and Grayed Out" ("禁用")) -> (error out=w255:errorcluster)  [unwired: 1 in, 1 out]
            n249 = property on="Close Device" class="Bool"(error in=w255, "DisabledEnum"=T7."Enabled" ("禁用")) -> (error out=w252:errorcluster)  [unwired: 1 in, 1 out]
            n250 = property on="Trigger Mode" class="Bool"(error in=w252, "DisabledEnum"=T7."Enabled" ("禁用")) -> (error out=w250:errorcluster)  [unwired: 1 in, 1 out]
            n251 = property on="Continuous" class="Bool"(error in=w250, "DisabledEnum"=T7."Disabled and Grayed Out" ("禁用")) -> (error out=w248:errorcluster)  [unwired: 1 in, 1 out]
            n252 = property on="打开标志" class="Bool (严格)"(error in=w248, "Value"=TRUE ("布尔")) -> ()  [unwired: 1 in, 2 out]
          }
          frame True {
            n253 = call "DestroyHandle.vi"("handle"=w263) -> ()  [unwired: 9 in, 2 out]
            n254 = One Button Dialog(message="Open Cam2 Failed") -> ()  [unwired: 1 in, 1 out]
            n255 = property on="打开标志" class="Bool (严格)"("Value"=FALSE) -> ()  [unwired: 2 in, 2 out]
          }
        }
      }
    }
    n256 = property on="handle out 2" class="DigNum (严格)"() -> ("Value"=w25:u64)  [unwired: 2 in, 2 out]
    n257 = case shown="真" "Close Device" {
      tunnel: w25 -> [_ w187]
      frame False {
      }
      frame True {
        n258 = call "CloseDevice.vi"("handle"=w187) -> ("error out"=w190:errorcluster, "handle out"=w188:u64)  [unwired: 8 in, 1 out]
        n259 = call "DestroyHandle.vi"("error in (no error)"=w190, "handle"=w188) -> ("error out"=w189:errorcluster)  [unwired: 8 in, 1 out]
        n260 = property on="Open Device" class="Bool"(error in=w189, "DisabledEnum"=T7."Enabled" ("禁用")) -> (error out=w203:errorcluster)  [unwired: 1 in, 1 out]
        n261 = property on="Close Device" class="Bool"(error in=w203, "DisabledEnum"=T7."Disabled and Grayed Out" ("禁用")) -> (error out=w202:errorcluster)  [unwired: 1 in, 1 out]
        n262 = property on="Start" class="Bool"(error in=w202, "DisabledEnum"=T7."Disabled and Grayed Out" ("禁用")) -> (error out=w201:errorcluster)  [unwired: 1 in, 1 out]
        n263 = property on="Stop" class="Bool"(error in=w201, "DisabledEnum"=T7."Disabled and Grayed Out" ("禁用")) -> (error out=w200:errorcluster)  [unwired: 1 in, 1 out]
        n264 = property on="Trigger Once" class="Bool"(error in=w200, "DisabledEnum"=T7."Disabled and Grayed Out" ("禁用")) -> (error out=w197:errorcluster)  [unwired: 1 in, 1 out]
        n265 = property on="Continuous" class="Bool"(error in=w197, "DisabledEnum"=T7."Disabled and Grayed Out" ("禁用")) -> (error out=w195:errorcluster)  [unwired: 1 in, 1 out]
        n266 = property on="Trigger Mode" class="Bool"(error in=w195, "DisabledEnum"=T7."Disabled and Grayed Out" ("禁用")) -> (error out=w194:errorcluster)  [unwired: 1 in, 1 out]
        n267 = property on="打开标志" class="Bool (严格)"(error in=w194, "Value"=FALSE ("打开标志")) -> (error out=w192:errorcluster)  [unwired: 1 in, 1 out]
        n268 = property on="Acquisision Flag" class="Bool (严格)"(error in=w192, "Value"=FALSE ("采集标志")) -> ()  [unwired: 1 in, 2 out]
      }
    }
    n269 = property on="handle out 2" class="DigNum (严格)"() -> ("Value"=w9:u64)  [unwired: 2 in, 2 out]
    n270 = property on="handle out" class="DigNum (严格)"() -> ("Value"=w43:u64)  [unwired: 2 in, 2 out]
  }
  n271 = property on="handle out" class="DigNum (严格)"() -> ("Value"=w3:u64)  [unwired: 2 in, 2 out]
  n272 = case shown="真" w5 {
    tunnel: w3 -> [_ w531]
    frame False {
    }
    frame True {
      n273 = property on="打开标志" class="Bool (严格)"() -> ("Value"=w522:bool)  [unwired: 2 in, 2 out]
      n274 = case shown="真" w522 {
        tunnel: w531 -> [_ w538]
        frame False {
        }
        frame True {
          n275 = call "CloseDevice.vi"("handle"=w538) -> ("error out"=w539:errorcluster, "handle out"=w537:u64)  [unwired: 8 in, 1 out]
          n276 = call "DestroyHandle.vi"("error in (no error)"=w539, "handle"=w537) -> ()  [unwired: 8 in, 2 out]
        }
      }
      n277 = property on="Open Device" class="Bool"("DisabledEnum"=T7."Enabled" ("禁用")) -> (error out=w530:errorcluster)  [unwired: 2 in, 1 out]
      n278 = property on="Close Device" class="Bool"(error in=w530, "DisabledEnum"=T7."Disabled and Grayed Out" ("禁用")) -> (error out=w529:errorcluster)  [unwired: 1 in, 1 out]
      n279 = property on="Trigger Once" class="Bool"(error in=w529, "DisabledEnum"=T7."Disabled and Grayed Out" ("禁用")) -> (error out=w528:errorcluster)  [unwired: 1 in, 1 out]
      n280 = property on="Start" class="Bool"(error in=w528, "DisabledEnum"=T7."Disabled and Grayed Out" ("禁用")) -> (error out=w527:errorcluster)  [unwired: 1 in, 1 out]
      n281 = property on="Stop" class="Bool"(error in=w527, "DisabledEnum"=T7."Disabled and Grayed Out" ("禁用")) -> (error out=w526:errorcluster)  [unwired: 1 in, 1 out]
      n282 = property on="Continuous" class="Bool"(error in=w526, "DisabledEnum"=T7."Disabled and Grayed Out" ("禁用")) -> (error out=w524:errorcluster)  [unwired: 1 in, 1 out]
      n283 = property on="Trigger Mode" class="Bool"(error in=w524, "DisabledEnum"=T7."Disabled and Grayed Out" ("禁用")) -> (error out=w519:errorcluster)  [unwired: 1 in, 1 out]
      n284 = property on="打开标志" class="Bool (严格)"(error in=w519, "Value"=FALSE ("打开标志")) -> (error out=w518:errorcluster)  [unwired: 1 in, 1 out]
      n285 = property on="Acquisision Flag" class="Bool (严格)"(error in=w518, "Value"=FALSE ("采集标志")) -> ()  [unwired: 1 in, 2 out]
    }
  }
  n286 = property on="handle out 2" class="DigNum (严格)"() -> ("Value"=w2:u64)  [unwired: 2 in, 2 out]
  n287 = case shown="真" w1 {
    tunnel: w2 -> [_ w553]
    frame False {
    }
    frame True {
      n288 = property on="打开标志" class="Bool (严格)"() -> ("Value"=w544:bool)  [unwired: 2 in, 2 out]
      n289 = case shown="真" w544 {
        tunnel: w553 -> [_ w560]
        frame False {
        }
        frame True {
          n290 = call "CloseDevice.vi"("handle"=w560) -> ("error out"=w561:errorcluster, "handle out"=w559:u64)  [unwired: 8 in, 1 out]
          n291 = call "DestroyHandle.vi"("error in (no error)"=w561, "handle"=w559) -> ()  [unwired: 8 in, 2 out]
        }
      }
      n292 = property on="Open Device" class="Bool"("DisabledEnum"=T7."Enabled" ("禁用")) -> (error out=w552:errorcluster)  [unwired: 2 in, 1 out]
      n293 = property on="Close Device" class="Bool"(error in=w552, "DisabledEnum"=T7."Disabled and Grayed Out" ("禁用")) -> (error out=w551:errorcluster)  [unwired: 1 in, 1 out]
      n294 = property on="Trigger Once" class="Bool"(error in=w551, "DisabledEnum"=T7."Disabled and Grayed Out" ("禁用")) -> (error out=w550:errorcluster)  [unwired: 1 in, 1 out]
      n295 = property on="Start" class="Bool"(error in=w550, "DisabledEnum"=T7."Disabled and Grayed Out" ("禁用")) -> (error out=w549:errorcluster)  [unwired: 1 in, 1 out]
      n296 = property on="Stop" class="Bool"(error in=w549, "DisabledEnum"=T7."Disabled and Grayed Out" ("禁用")) -> (error out=w548:errorcluster)  [unwired: 1 in, 1 out]
      n297 = property on="Continuous" class="Bool"(error in=w548, "DisabledEnum"=T7."Disabled and Grayed Out" ("禁用")) -> (error out=w546:errorcluster)  [unwired: 1 in, 1 out]
      n298 = property on="Trigger Mode" class="Bool"(error in=w546, "DisabledEnum"=T7."Disabled and Grayed Out" ("禁用")) -> (error out=w541:errorcluster)  [unwired: 1 in, 1 out]
      n299 = property on="打开标志" class="Bool (严格)"(error in=w541, "Value"=FALSE ("打开标志")) -> (error out=w540:errorcluster)  [unwired: 1 in, 1 out]
      n300 = property on="Acquisision Flag" class="Bool (严格)"(error in=w540, "Value"=FALSE ("采集标志")) -> ()  [unwired: 1 in, 2 out]
    }
  }
